vi "Save Plugin setups Question.vi"(0 "VI path":path) -> (1 "Load Plugin Setup":bool, 2 "Save Plugin Setup":bool, 3 "Plugin_Label":string)   [LabVIEW 2022 SP3]
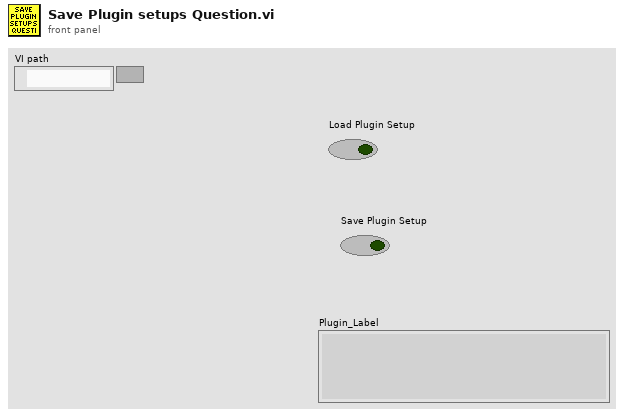
[diagram p1: front panel]
types:
  T1 = enum32{"Bad", "Idle", "Run top level", "Running"}
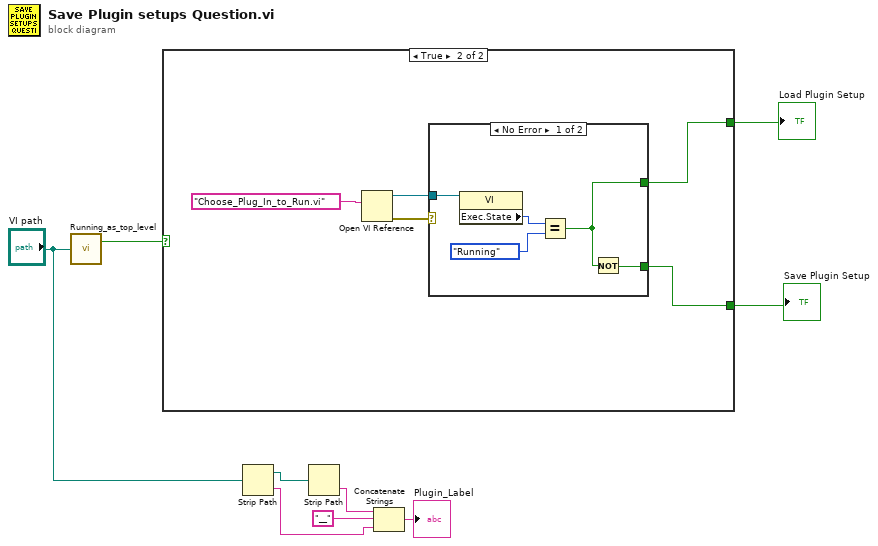
[diagram p0: block diagram]
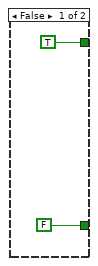
[diagram p2: hidden frame]
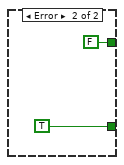
[diagram p3: hidden frame]
diagram:
  n1 = call "Running_as_top_level.vi"("Vi path name"="VI path") -> ("Top Level"=w9:bool)  [unwired: 1 out]
  n2 = case shown="True" w9 {
    tunnel: [TRUE w12] -> w8
    tunnel: [FALSE w13] -> w7
    frame False {
    }
    frame True {
      n3 = Open VI Reference(vi path="Choose_Plug_In_to_Run.vi") -> (vi reference=w16:refnum<vi>, error out=w14:errorcluster)  [unwired: 5 in]
      n4 = case shown="No Error" w14 {
        tunnel: w16 -> [w21 _]
        tunnel: [w18 TRUE] -> w13
        tunnel: [w17 FALSE] -> w12
        frame No Error {
          n5 = property class="VI"(reference=w21) -> ("Exec.State"=w20:T1)  [unwired: 1 in, 2 out]
          n6 = Equal?(x=w20, y=T1."Running" ("Execution:State")) -> (x = y?=w17:bool)
          n7 = Not(x=w17) -> (.not. x?=w18:bool)
        }
        frame Error {
        }
      }
    }
  }
  "Load Plugin Setup" <- w8
  "Save Plugin Setup" <- w7
  n8 = Strip Path(path="VI path") -> (stripped path=w3:path, name=w5:string)
  n9 = Strip Path(path=w3) -> (name=w4:string)  [unwired: 1 out]
  n10 = Concatenate Strings(w4, "__" ("string"), w5) -> (→"Plugin_Label":string)
